vi "Own_Code_PS.vi"() -> ()   [LabVIEW 2012]
uses:
  SubVIs/LVPresent_Globals.vi
panel:
  in  "Tab Control":enum32{"Page 1", "Page 2"}(tab)
  in  "Open":bool
  in  "Need a hint/solution":bool
  in  "While Loop":bool
  in  "For Loop":bool
  in  "Step 2":bool
  in  "Step 1":bool
  in  "Back":bool
  # "Now it's your turn!\n\nNow that you've run through some code, let's try and write some of our own. We can start with something simple like turning on the red LED at the bottom of the Protosnap board (again, the RGB LEDs have opposite LO/HI commands than the other LEDs). Click the Open button to start a new VI. Can't find BotSpeak or open the functions palette? Check out the help! Also, for now it would probably be easier to leave on AutoTooling."
  # "Step 2:\n\nAfter you get the code running and the lights working, try making it shut off after a certain amount of time. This is very similar to the example completed earlier in the tutorial."
  # "Step 3:\n\nNow that your light turns on and off, try making it blink 5 times. Let's also have a case where it blinks forever."
  # "Check out the hints!"
  # "Hint 1: Start with a write command, as you will want the light to be outputting information. Also, the red LED is on pin 3. Remember, if you need help check out the menu in the bottom left corner.\n\n\n\nHint 2: You're definitely going to have to wait... \n\n\n\n\nHint 3: One case will require a For Loop, and the other will require a While Loop.\n\n\n\n\n\nHelpful Tip: When creating a constant, you can simply right click on the terminal you wish to wire to, click create-->constant. Note that constants aren't always necessarily numbers."
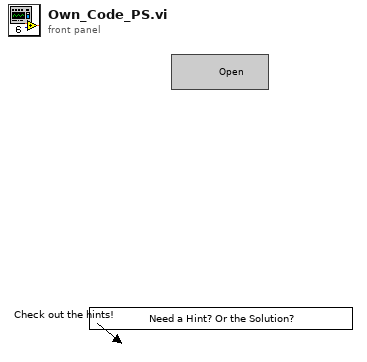
[diagram p1: front panel]
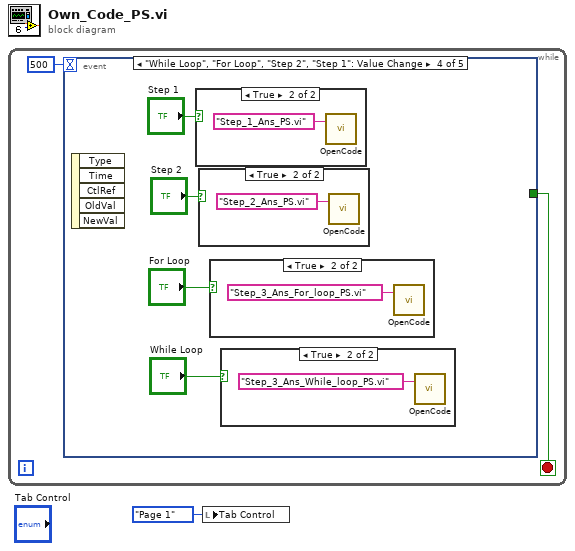
[diagram p0: block diagram]
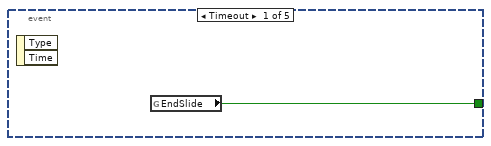
[diagram p2: hidden frame]
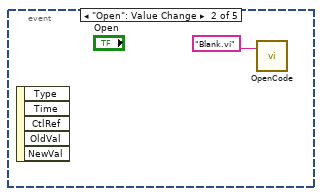
[diagram p3: hidden frame]
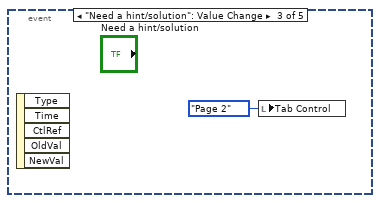
[diagram p4: hidden frame]
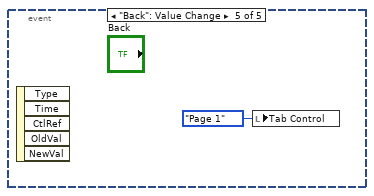
[diagram p9: hidden frame]
diagram:
  n1 = while {
    stop <- w3 stop-if-true
    n2 = event shown="[3] \"While Loop\", \"For Loop\", \"Step 2\", \"Step 1\": Value Change" {
      selector: _ -> [_ _ _ _ _]
      dyn-events: _ -> [_ _ _ _ _]
      timeout: 500 -> [_ _ _ _ _]
      tunnel: [w4 _ _ _ _] -> w3
      event Timeout {
        n3 = event-data() -> ()  [unwired: 1 in, 2 out]
        n4 = global read "LVPresent_Globals.vi" "EndSlide"() -> (w4:bool)
      }
      event "Open": Value Change {
        n5 = event-data() -> ()  [unwired: 1 in, 5 out]
        n6 = call "OpenCode.vi"("Code name"="Blank.vi") -> ()  [unwired: 3 in]
      }
      event "Need a hint/solution": Value Change {
        n7 = event-data() -> ()  [unwired: 1 in, 5 out]
        n8 = local write "Tab Control"(enum32{"Page 1", "Page 2"}."Page 2" ("Tab Control")) -> ()
      }
      event "While Loop", "For Loop", "Step 2", "Step 1": Value Change {
        n9 = event-data() -> ()  [unwired: 1 in, 5 out]
        n10 = case shown="True" "Step 1" {
          frame False {
          }
          frame True {
            n11 = call "OpenCode.vi"("Code name"="Step_1_Ans_PS.vi") -> ()  [unwired: 3 in]
          }
        }
        n12 = case shown="True" "Step 2" {
          frame False {
          }
          frame True {
            n13 = call "OpenCode.vi"("Code name"="Step_2_Ans_PS.vi") -> ()  [unwired: 3 in]
          }
        }
        n14 = case shown="True" "For Loop" {
          frame False {
          }
          frame True {
            n15 = call "OpenCode.vi"("Code name"="Step_3_Ans_For_loop_PS.vi") -> ()  [unwired: 3 in]
          }
        }
        n16 = case shown="True" "While Loop" {
          frame False {
          }
          frame True {
            n17 = call "OpenCode.vi"("Code name"="Step_3_Ans_While_loop_PS.vi") -> ()  [unwired: 3 in]
          }
        }
      }
      event "Back": Value Change {
        n18 = event-data() -> ()  [unwired: 1 in, 5 out]
        n19 = local write "Tab Control"(enum32{"Page 1", "Page 2"}."Page 1" ("Tab Control")) -> ()
      }
    }
  }
  n20 = local write "Tab Control"(enum32{"Page 1", "Page 2"}."Page 1" ("Tab Control")) -> ()
